vi "open_erg.vi"(3 "error in (no error)":errorcluster, 4 "baud rate":u32=19200, 5 "VISA resource name":refnum<visa-resource-name>) -> (0 "error out":errorcluster, 1 "Errors":bool, 2 "VISA resource name out":refnum<visa-resource-name>)   [LabVIEW 2018]
uses:
  <vilib>/Instr/_visa.llb/VISA Configure Serial Port (Instr).vi
panel:
  out "unsigned byte array":u8[](array[numeric])
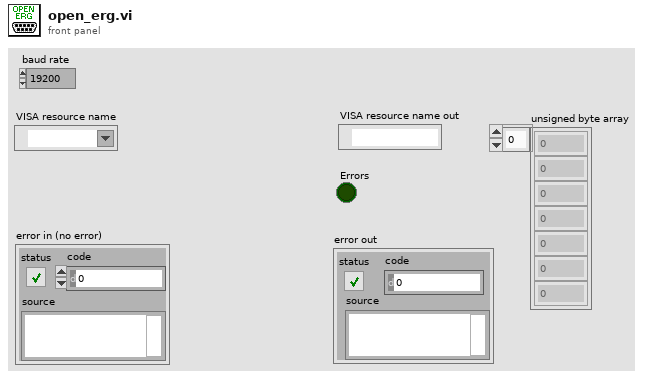
[diagram p1: front panel]
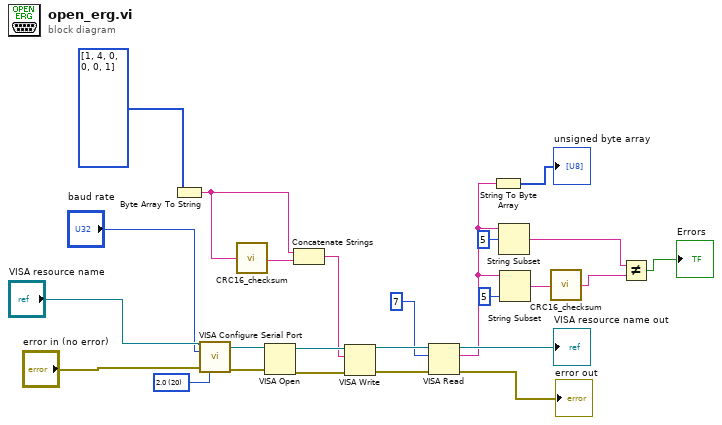
[diagram p0: block diagram]
diagram:
  w25 = u16 20 items=["1.0"=10, "1.5"=15, "2.0"=20] ("stop bits (10: 1 bit)")
  n1 = Byte Array To String(unsigned byte array=u8[] [1, 4, 0, 0, 0, 1]) -> (string=w16:string)
  n2 = call-poly "VISA Configure Serial Port"("VISA resource name"="VISA resource name", "baud rate (9600)"="baud rate", "error in (no error)"="error in (no error)", "stop bits (10: 1 bit)"=w25) -> ("VISA resource name out"=w23:refnum<visa-resource-name>, "error out"=w24:errorcluster)  [unwired: 10 in]
  n3 = call "CRC16_checksum.vi"("message"=w16) -> ("CRC16"=w17:string)
  n4 = VISA Open(error in (no error)=w24, VISA resource name=w23) -> (VISA resource name=w18:refnum<visa-resource-name>, error out=w19:errorcluster)  [unwired: 3 in]
  n5 = Concatenate Strings(w16, w17) -> (w15:string)
  n6 = VISA Write(VISA resource name=w18, write buffer=w15, error in (no error)=w19) -> (VISA resource name out=w12:refnum<visa-resource-name>, error out=w13:errorcluster)  [unwired: 1 out]
  n7 = VISA Read(VISA resource name=w12, byte count=u32 7, error in (no error)=w13) -> (VISA resource name out=→"VISA resource name out":refnum<visa-resource-name>, read buffer=w2:string, error out=→"error out":errorcluster)  [unwired: 1 out]
  n8 = String To Byte Array(string=w2) -> (unsigned byte array=→"unsigned byte array":u8[])
  n9 = String Subset(string=w2, offset (0)=5) -> (substring=w4:string)  [unwired: 1 in]
  n10 = String Subset(string=w2, length (rest)=5 ("length (rest)")) -> (substring=w6:string)  [unwired: 1 in]
  n11 = call "CRC16_checksum.vi"("message"=w6) -> ("CRC16"=w5:string)
  n12 = Not Equal?(x=w4, y=w5) -> (x != y?=→"Errors":bool)
